vi "GET Row.vi"(8 "Error in":errorcluster caption="Error in (no error)", 10 "Row ID":u32=701, 11 "Table ID":u32=701) -> (0 "Error out":errorcluster, 3 "Rows Array JSON":string)   [LabVIEW 2018]
uses:
  Attach Param - Bool.vi
  <vilib>/httpClient/LabVIEWHTTPClient.lvlib
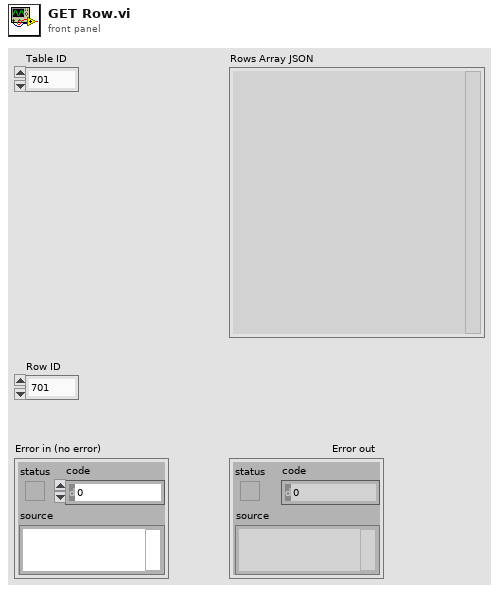
[diagram p1: front panel]
types:
  T1 = typedef "LabVIEWHTTPClient.lvlib/ClientHandle.ctl" = refnum<k1>
  T2 = typedef "Param.ctl" = cluster{"Param":string, "Value":string}
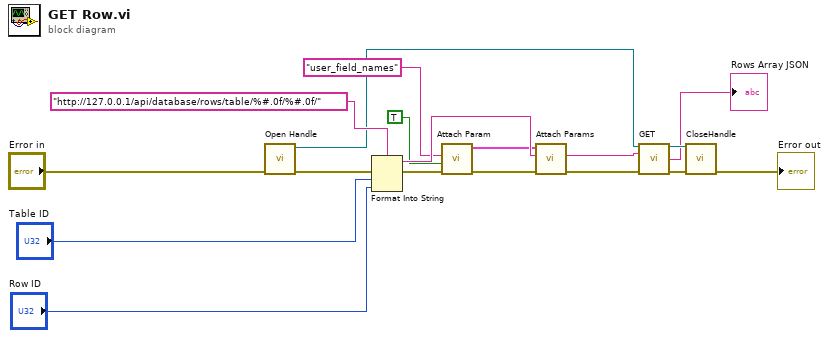
[diagram p0: block diagram]
diagram:
  n1 = call "Open Handle.vi"("error in (no error)"="Error in") -> ("error out"=w14:errorcluster, "Refnum out"=w13:T1)  [unwired: 9 in]
  n2 = Format Into String(format string="http://127.0.0.1/api/database/rows/table/%#.0f/%#.0f/" ("url"), error in=w14, "Table ID", "Row ID") -> (resulting string=w18:string, error out=w8:errorcluster)  [unwired: 1 in]
  n3 = call-poly "Attach Param.vi"("Error in"=w8, "Value"=TRUE, "Param Name"="user_field_names") -> ("Error out"=w3:errorcluster, "Params Array Out"=w4:T2[])  [unwired: 7 in]
  n4 = call "Attach Params.vi"("Error in"=w3, "URL"=w18, "Param array"=w4) -> ("Error out"=w5:errorcluster, "URL with params"=w6:string)  [unwired: 7 in]
  n5 = call <vilib>:"GET.vi"("client handle"=w13, "url"=w6, "error in (no error)"=w5) -> ("client handle out"=w15:T1, "body"=→"Rows Array JSON":string, "error out"=w1:errorcluster)  [unwired: 9 in, 1 out]
  n6 = call <vilib>:"CloseHandle.vi"("client handle"=w15, "error in (no error)"=w1) -> ("error out"=→"Error out":errorcluster)  [unwired: 13 in]
